vi "Check Status.vi"(0 "VISA resource name":refnum<visa-resource-name>, 11 "error in (no error)":errorcluster) -> (4 "VISA resource name out":refnum<visa-resource-name>, 15 "error out":errorcluster)   [LabVIEW 2012, in "Fluke 5XXX Series Multicalibrators.lvlib"]
doc: "This VI reads the Standard Event Register and checks it for error. When Error occured, use Error Query VI to describe error type."
uses:
  Fluke 5XXX Series Multicalibrators.lvlib
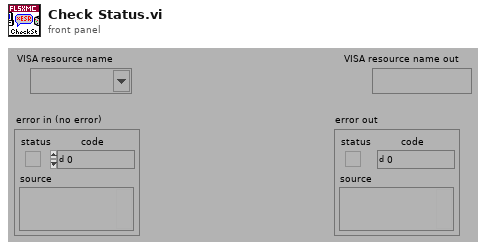
[diagram p1: front panel]
types:
  T1 = cluster{"Status":bool, "Code":i32, "Source (VI Name)":string}
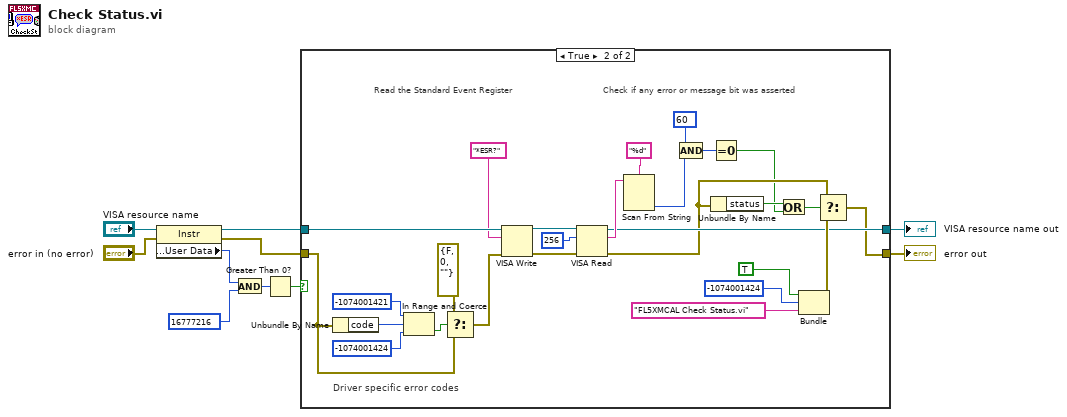
[diagram p0: block diagram]
diagram:
  n1 = property class="Instr"(reference="VISA resource name", error in="error in (no error)") -> (reference out=w7:refnum<visa-resource-name>, error out=w6:errorcluster, "General Settings:User Data"=w4:u32)
  n2 = And(x=w4, y=u32 16777216) -> (x .and. y?=w2:u32)
  n3 = Greater Than 0?(x=w2) -> (x > 0?=w1:bool)
  n4 = case shown="True" w1 {
    tunnel: w6 -> [w12 w15]
    tunnel: w7 -> [w11 w39]
    tunnel: [w11 w23] -> w10
    tunnel: [w12 w21] -> w9
    frame False {
    }
    frame True {
      # "Driver specific error codes"
      # "Check if any error or message bit was asserted"
      # "Read the Standard Event Register"
      n5 = Unbundle By Name(w15) -> ("code"=w18:i32)
      n6 = In Range and Coerce(upper limit=-1074001421, x=w18, lower limit=-1074001424) -> (In Range?=w19:bool)  [unwired: 1 out]
      n7 = Select(t=errorcluster {"status"=FALSE, "code"=0, "source"=""} ("error out"), s=w19, f=w15) -> (s? t:f=w14:errorcluster)
      n8 = VISA Write(VISA resource name=w39, write buffer="*ESR?", error in (no error)=w14) -> (VISA resource name out=w35:refnum<visa-resource-name>, error out=w34:errorcluster)  [unwired: 1 out]
      n9 = VISA Read(VISA resource name=w35, byte count=u32 256 ("byte count (0)"), error in (no error)=w34) -> (VISA resource name out=w23:refnum<visa-resource-name>, read buffer=w32:string, error out=w22:errorcluster)  [unwired: 1 out]
      n10 = Scan From String(format string="%d", input string=w32) -> (output 1=w31:i32)  [unwired: 3 in, 3 out]
      n11 = Compound Arithmetic op=AND(60 ("status"), w31) -> (w36:i32)
      n12 = Equal To 0?(x=w36) -> (x = 0?=w13:bool)
      n13 = Unbundle By Name(w22) -> ("status"=w27:bool)
      n14 = Or(x=w27, y=w13) -> (x .or. y?=w28:bool)
      n15 = Bundle("Status"=TRUE, "Code"=-1074001424, "Source (VI Name)"="FL5XMCAL Check Status.vi") -> (w26:T1)  [unwired: 1 in]
      n16 = Select(t=w22, s=w28, f=w26) -> (s? t:f=w21:T1)
    }
  }
  "error out" <- w9
  "VISA resource name out" <- w10
